vi "Single Video Display1.vi"() -> ()   [LabVIEW 2017]
uses:
  VideoWindowsCommand.ctl
  <vilib>/Utility/miscctls.llb/LVPositionTypeDef.ctl
  <vilib>/Utility/config.llb/NI_LVConfig.lvlib
panel:
  out "string":string
  out "path":path
  in  "Video Feed":enum16{"Camera 1", "Camera2", "Mobile"}(ring)=enum."Camera2"
  in  "MozillaBrowser 2":refnum<k7>(container)
  in  "Exit":bool
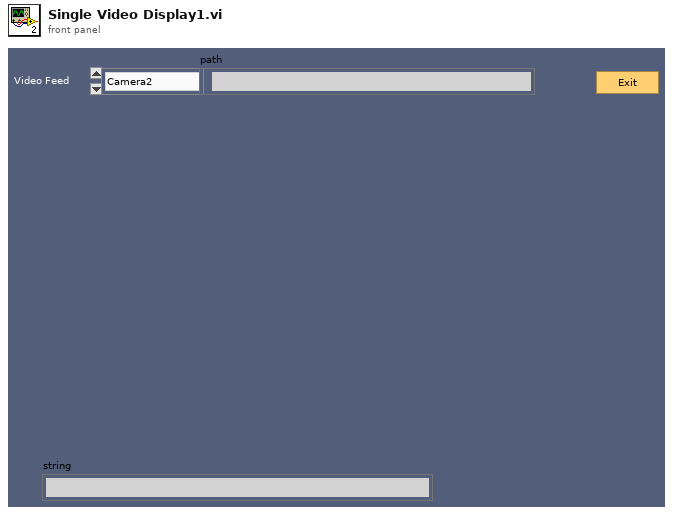
[diagram p1: front panel]
types:
  T1 = typedef "NI_LVConfig.lvlib/Config Data RefNum.ctl" = refnum<k1>
  T2 = typedef "VideoWindowsCommand.ctl" = cluster{"Position":T3, "Exit":bool, "MoveToFront":bool}
  T3 = typedef "LVPositionTypeDef.ctl" = cluster{"Left":i32, "Top":i32}
  T4 = typedef "LVRectTypeDef.ctl" = cluster{"Left":i16, "Top":i16, "Right":i16, "Bottom":i16}
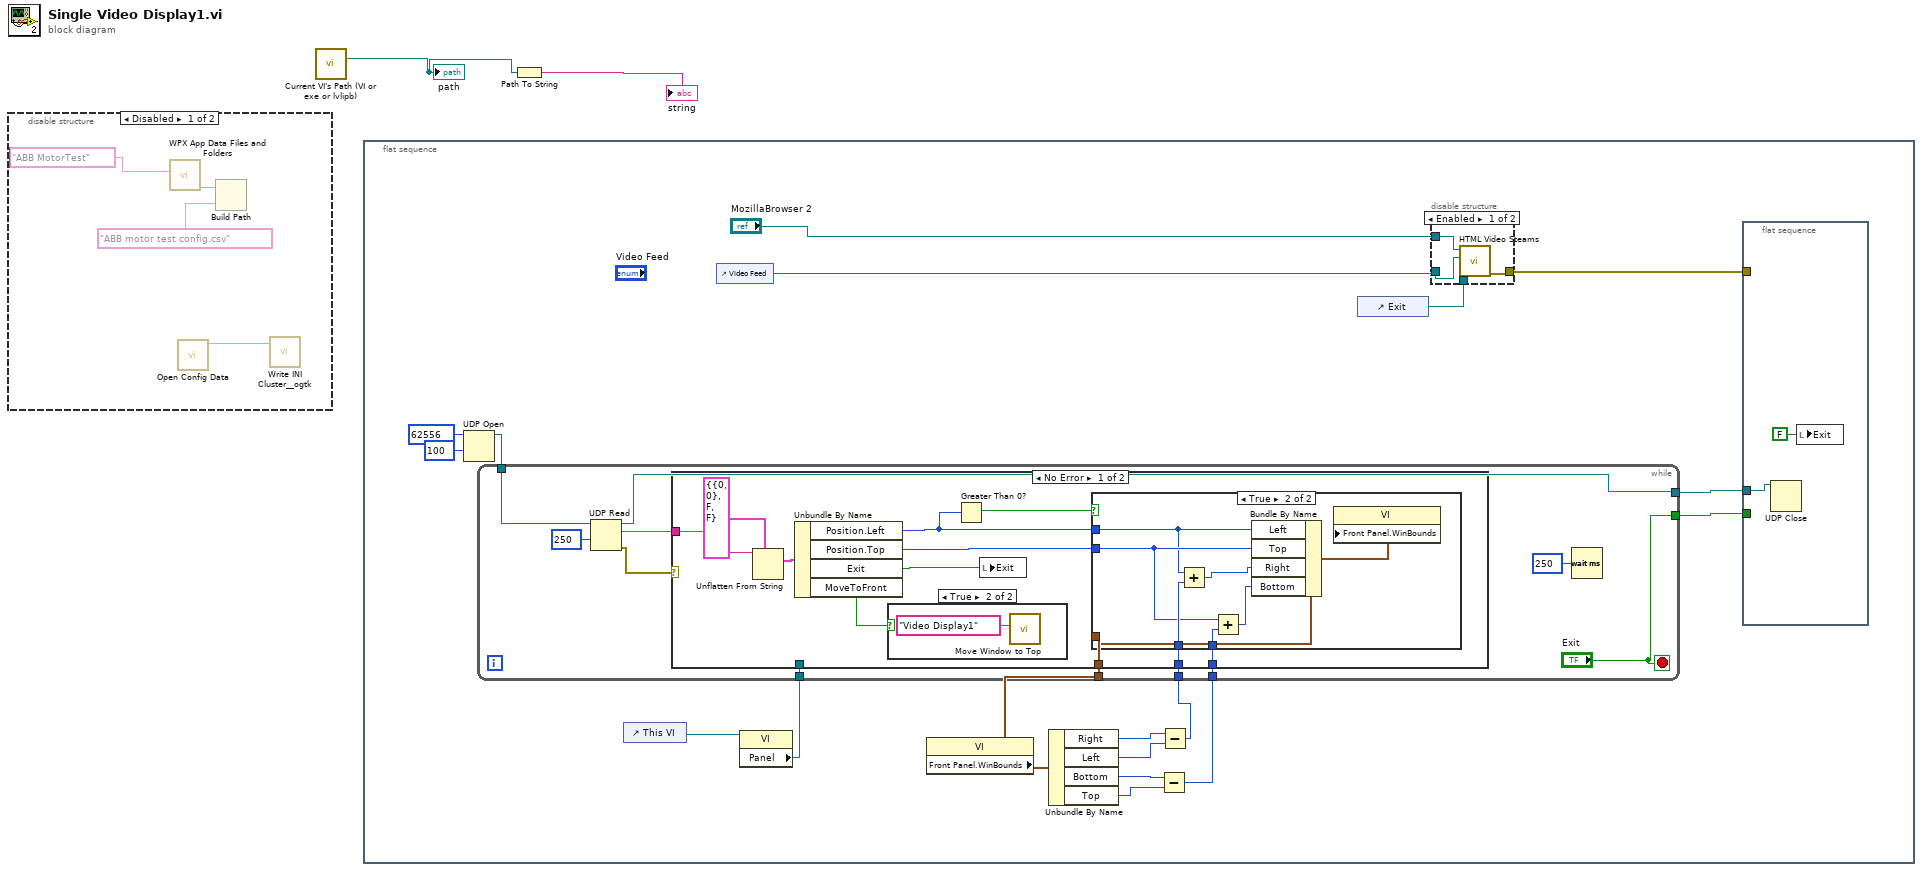
[diagram p0: block diagram]
diagram:
  n1 = disable-structure shown="Disabled" {
    frame Disabled {
      n2 = call "WPX App Data Files and Folders.vi"("ApplicationName"="ABB MotorTest") -> ("DataFolder"=w3:path)  [unwired: 7 in, 3 out]
      n3 = call <vilib>:"Open Config Data.vi"() -> ("refnum"=w6:T1)  [unwired: 9 in, 2 out]
      n4 = Build Path(base path=w3, name or relative path="ABB motor test config.csv") -> ()  [unwired: 1 out]
      n5 = call <userlib>:"Write INI Cluster__ogtk.vi"("refnum"=w6) -> ()  [unwired: 9 in, 2 out]
    }
    frame Enabled {
    }
  }
  n6 = call "Current VI's Path (VI or exe or lvlipb).vi"() -> ("Full Path to VI or executable"=w1:path)  [unwired: 14 in, 1 out]
  "path" <- w1
  n7 = flat-sequence {
    frame #0 {
      n8 = UDP Open(9:100 ("timeout ms (25000)"), 11:u16 62556 ("port")) -> (port=w19:refnum<k16>)  [unwired: 3 in, 2 out]
      n9 = control-ref of="This VI"() -> (w18:refnum<vi>)
      n10 = control-ref of="Video Feed"() -> (w23:refnum<vi>)
      n11 = property class="VI"(reference=w18) -> ("Panel"=w17:refnum<vi>)  [unwired: 1 in, 2 out]
      n12 = property class="VI"() -> ("Front Panel.WinBounds"=w10:T4)  [unwired: 2 in, 2 out]
      n13 = Unbundle By Name(w10) -> ("Right"=w13:i16, "Left"=w14:i16, "Bottom"=w11:i16, "Top"=w12:i16)
      n14 = Subtract(x=w11, y=w12) -> (x-y=w8:i16)
      n15 = Subtract(x=w13, y=w14) -> (x-y=w9:i16)
      n16 = while {
        tunnel: ["Exit"] -> w21
        tunnel: w19 -> [w35]
        tunnel: w17 -> [w31]
        tunnel: [w30] -> w16
        tunnel: w10 -> [w29]
        tunnel: w9 -> [w28]
        tunnel: w8 -> [w27]
        stop <- "Exit" stop-if-true
        n17 = UDP Read(connection ID=w35, timeout ms (25000)=250) -> (data out=w32:string, error out=w33:errorcluster, 3:w30:refnum<k16>)  [unwired: 2 in, 2 out]
        n18 = case shown="No Error" w33 {
          tunnel: w32 -> [w48 _]
          tunnel: w31 -> [_ _]
          tunnel: w29 -> [w44 _]
          tunnel: w28 -> [w43 _]
          tunnel: w27 -> [w41 _]
          frame No Error {
            n19 = Unflatten From String(type=T2 {"Position"={"Left"=0, "Top"=0}, "Exit"=FALSE, "MoveToFront"=FALSE}, binary string=w48) -> (value=w46:T2)  [unwired: 3 in, 2 out]
            n20 = Unbundle By Name(w46) -> ("Position.Left"=w40:i32, "Position.Top"=w42:i32, "Exit"=w45:bool, "MoveToFront"=w38:bool)
            n21 = case shown="True" w38 {
              frame False {
              }
              frame True {
                n22 = call "Move Window to Top.vi"("window name (\"\")"="Video Display1" ("window name (\"\")")) -> ()  [unwired: 5 in, 2 out]
              }
            }
            n23 = Greater Than 0?(x=w40) -> (x > 0?=w39:bool)
            n24 = local write "Exit"(w45) -> ()
            n25 = case shown="True" w39 {
              tunnel: w44 -> [_ w57]
              tunnel: w43 -> [_ w56]
              tunnel: w42 -> [_ w54]
              tunnel: w41 -> [_ w53]
              tunnel: w40 -> [_ w50]
              frame False {
              }
              frame True {
                n26 = Add(x=w50, y=w56) -> (x+y=w55:i32)
                n27 = Add(x=w54, y=w53) -> (x+y=w52:i32)
                n28 = Bundle By Name(cluster=w57, "Left"=w50, "Top"=w54, "Right"=w55, "Bottom"=w52) -> (w51:T4)
                n29 = property class="VI"("Front Panel.WinBounds"=w51) -> ()  [unwired: 2 in, 2 out]
              }
            }
          }
          frame Error {
          }
        }
        n30 = Wait (ms)(milliseconds to wait=u32 250) -> ()  [unwired: 1 out]
      }
      n31 = control-ref of="Exit"() -> (w7:refnum<vi>)
      n32 = disable-structure shown="Enabled" {
        disable-tunnel: "MozillaBrowser 2" -> [w61 _]
        disable-tunnel: w23 -> [w60 _]
        disable-tunnel: [w59 _] -> w22
        disable-tunnel: w7 -> [w58 _]
        frame Enabled {
          n33 = call "HTML Video Steams.vi"("Exit"=w58, "Video Feed 2"=w60, "Automation Refnum in"=w61) -> ("error out"=w59:errorcluster)  [unwired: 7 in, 1 out]
        }
        frame Disabled {
        }
      }
      n34 = flat-sequence {
        tunnel: w22 -> [_]
        tunnel: w21 -> [_]
        tunnel: w16 -> [w25]
        frame #0 {
          n35 = UDP Close(connection ID=w25) -> ()  [unwired: 1 in, 2 out]
          n36 = local write "Exit"(FALSE ("Exit")) -> ()
        }
      }
    }
  }
  n37 = Path To String(path=w1) -> (string=→"string":string)
